vi "Rule Base Chart and Fault Probabilites Ver001.vi"(6 "s - value":dbl=1.0, 8 "Feature Thresholds":dbl[](array[numeric])=[0.583, 0.9072, 1.361, 0.43, 0.743, 0.346, 0.493], 9 "Rule Array":dbl[][](array[numeric])=[[1.0, 0.0, 1.0, -1.0, -1.0, -1.0, -1.0], [1.0, 0.0, 1.0, 1.0, -1.0, 0.0, -1.0], [-1.0, 0.0, 0.0, -1.0, 0.0, -1.0, 1.0], [-1.0, 1.0, 1.0, -1.0, 1.0, -1.0, -1.0], [0.0, 0.0, 0.0, -1.0, -1.0, -1.0, -1.0], [0.0, 0.0, 1.0, 1.0, 1.0, 0.0, 0.0], [0.0, 0.0, 0.0, 0.0, 0.0, 0.0, 0.0]], 10 "Predicted Values":dbl[](array[numeric]), 11 "Measured Values":dbl[](array[numeric])) -> (0 "Individual Probabilities (0>1)":dbl[][](array[numeric])=[[1.0, 0.0, 1.0, -1.0, -1.0, -1.0, -1.0], [1.0, 0.0, 1.0, 1.0, -1.0, 0.0, -1.0], [-1.0, 0.0, 0.0, -1.0, 0.0, -1.0, 1.0], [-1.0, 1.0, 1.0, -1.0, 1.0, -1.0, -1.0], [0.0, 0.0, 0.0, -1.0, -1.0, -1.0, -1.0], [0.0, 0.0, 1.0, 1.0, 1.0, 0.0, 0.0], [0.0, 0.0, 0.0, 0.0, 0.0, 0.0, 0.0]] format="%.2f", 1 "Fault Probability":dbl[](array[numeric]) format="%.4e", 2 "Neutral, Negative, Positive":dbl[][](array[numeric]) format="%.3e", 3 "Residuals":dbl[](array[numeric]), 4 "Individual Probabilities (%)":dbl[][](array[numeric])=[[1.0, 0.0, 1.0, -1.0, -1.0, -1.0, -1.0], [1.0, 0.0, 1.0, 1.0, -1.0, 0.0, -1.0], [-1.0, 0.0, 0.0, -1.0, 0.0, -1.0, 1.0], [-1.0, 1.0, 1.0, -1.0, 1.0, -1.0, -1.0], [0.0, 0.0, 0.0, -1.0, -1.0, -1.0, -1.0], [0.0, 0.0, 1.0, 1.0, 1.0, 0.0, 0.0], [0.0, 0.0, 0.0, 0.0, 0.0, 0.0, 0.0]] format="%.2f")   [LabVIEW 2017]
panel:
  in  "Tab Control":T1(tab)
  out "Sum of Probs":dbl[](array[numeric]) format="%_2f"
  # "Rule Based Chart"
  # "Te"
  # "Tsh"
  # "TD"
  # "Order\nfrom top\nto bottom\nas seen in\nTable 5.2 \n(Left to right)"
  # "TC"
  # "Tsc"
  # "dTCA"
  # "dTEA"
  # "Te"
  # "Tsh"
  # "TD"
  # "TC"
  # "Tsc"
  # "dTCA"
  # "dTEA"
  # "Tsh"
  # "TD"
  # "TC"
  # "Tsc"
  # "dTCA"
  # "Te"
  # "dTEA"
  # "CMF = Comp Valve Leakage"
  # "ODFoul = OD Coil Fouling"
  # "IDFoul = ID Coil Fouling"
  # "LL = Liq. Line Restriction"
  # "UC = Undercharge (- %)"
  # "OC = Overcharge (+ %)"
  # "NF = No Fault"
  # "Te"
  # "Tsh"
  # "TD"
  # "TC"
  # "Tsc"
  # "dTCA"
  # "dTEA"
  # "0"
  # "-1"
  # "1"
  # "CMF = Comp Valve Leakage"
  # "ODFoul = OD Coil Fouling"
  # "IDFoul = ID Coil Fouling"
  # "LL = Liq. Line Restriction"
  # "UC = Undercharge (- %)"
  # "OC = Overcharge (+ %)"
  # "NF = No Fault"
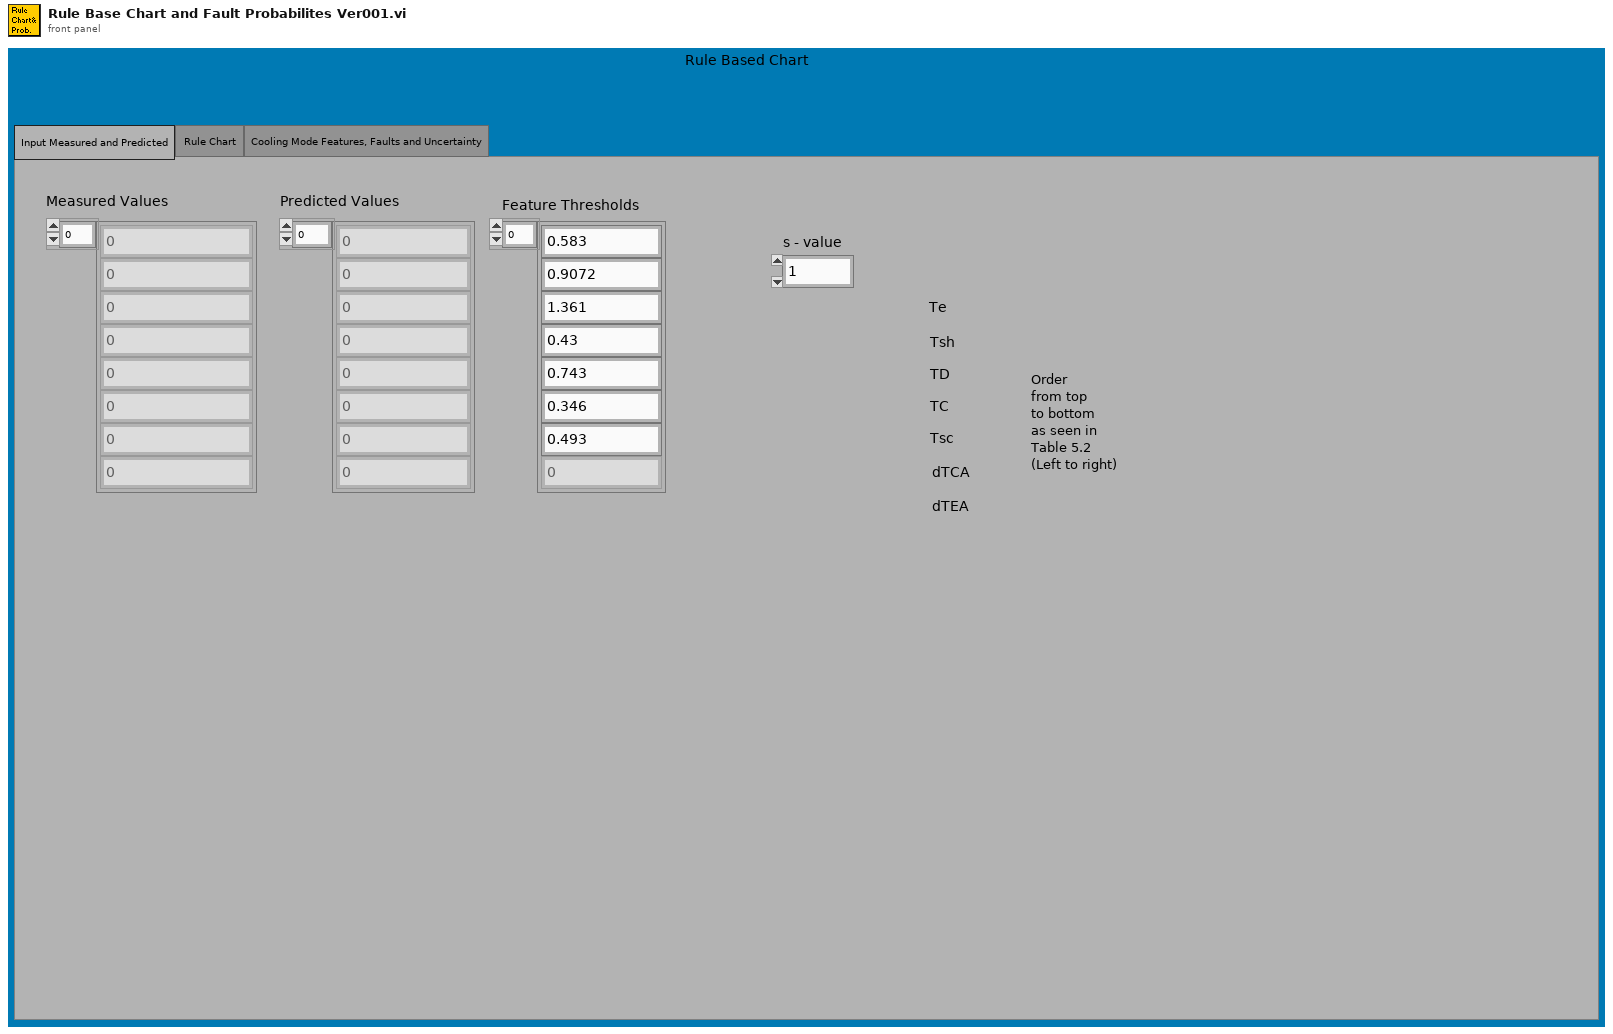
[diagram p1: front panel]
types:
  T1 = enum32{"Input Measured and Predicted", "Rule Chart ", "Cooling Mode Features, Faults and Uncertainty"}
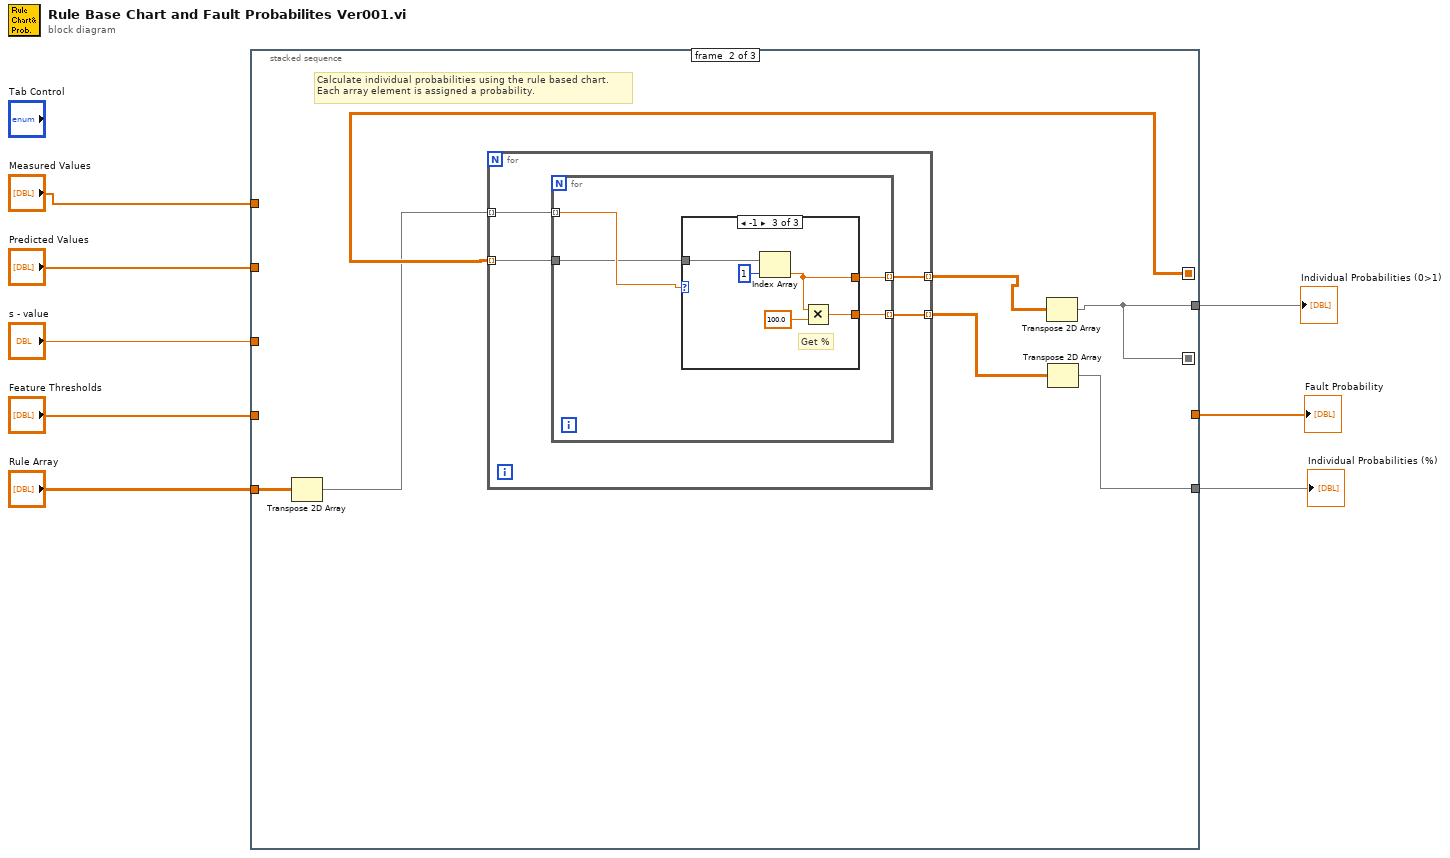
[diagram p0: block diagram]
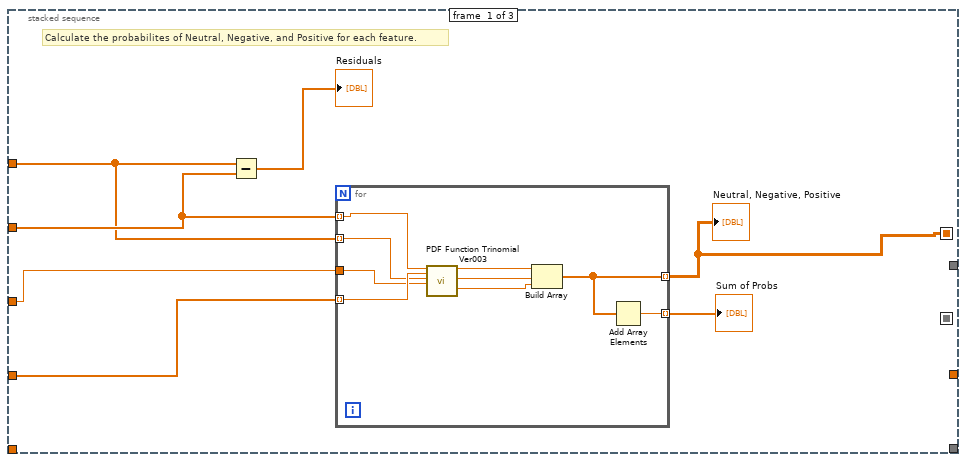
[diagram p2: hidden frame]
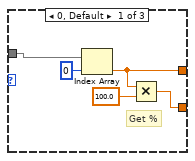
[diagram p3: hidden frame]
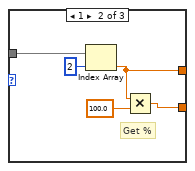
[diagram p4: hidden frame]
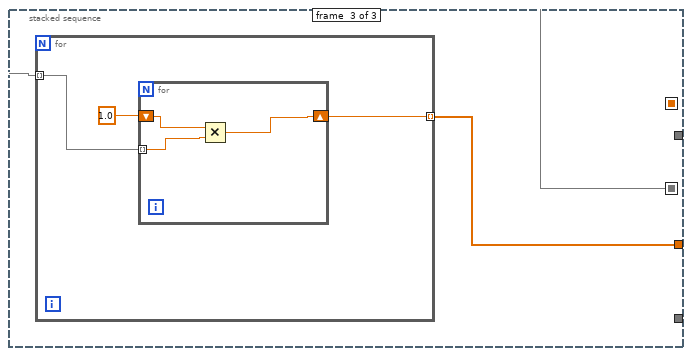
[diagram p5: hidden frame]
diagram:
  n1 = stacked-sequence {
    seq-local: [w9 _ _] -> [_ w31 _]
    seq-local: [_ w27 _] -> [_ _ w56]
    tunnel: "Measured Values" -> [w13 _ _]
    tunnel: "Predicted Values" -> [w14 _ _]
    tunnel: "s - value" -> [w12 _ _]
    tunnel: "Feature Thresholds" -> [w11 _ _]
    tunnel: "Rule Array" -> [_ w30 _]
    tunnel: [_ w27 _] -> w3
    tunnel: [_ _ w55] -> w2
    tunnel: [_ w25 _] -> w1
    frame #0 {
      # "Calculate the probabilites of Neutral, Negative, and Positive for each feature."
      n2 = Subtract(x=w13, y=w14) -> (x-y=→"Residuals":dbl[])
      n3 = for {
        tunnel: w14 -> [w24] mode=indexing
        tunnel: w13 -> [w22] mode=indexing
        tunnel: w12 -> [w21]
        tunnel: w11 -> [w23] mode=indexing
        tunnel: [w17] -> w9 mode=indexing
        tunnel: [w16] -> w10 mode=indexing
        n4 = call "PDF Function Trinomial Ver003.vi"("NFSS Ref \nModel Value"=w24, "NFSS Ref Std Dev"=w23, "Current Measured Value\nor Moving Window Mean"=w22, "s - value"=w21) -> ("Probability of NEUTRAL"=w20:dbl, "Prob NEGATIVE\nor DECREASING"=w19:dbl, "Prob POSITIVE\nor INCREASING"=w18:dbl)  [unwired: 13 out]
        n5 = Build Array(w20, w19, w18) -> (w17:dbl[])
        n6 = Add Array Elements(numeric array=w17) -> (sum=w16:dbl)
      }
      "Neutral, Negative, Positive" <- w9
      "Sum of Probs" <- w10
    }
    frame #1 {
      # "Calculate individual probabilities using the rule based chart.\nEach array element is assigned a probability."
      n7 = Transpose 2D Array(2D array=w30) -> (transposed array=w29:dbl[][])
      n8 = for {
        tunnel: w29 -> [w35] mode=indexing
        tunnel: w31 -> [w34] mode=indexing
        tunnel: [w33] -> w28 mode=indexing
        tunnel: [w32] -> w26 mode=indexing
        n9 = for {
          tunnel: w35 -> [w39] mode=indexing
          tunnel: w34 -> [w38]
          tunnel: [w37] -> w33 mode=indexing
          tunnel: [w36] -> w32 mode=indexing
          n10 = case shown="-1" w39 {
            tunnel: w38 -> [w44 w48 w53]
            tunnel: [w41 w46 w51] -> w37
            tunnel: [w40 w45 w50] -> w36
            frame 0, Default {
              # "Get %"
              n11 = Index Array(array=w44, index=0) -> (element=w41:dbl)
              n12 = Multiply(x=w41, y=100.0) -> (x*y=w40:dbl)
            }
            frame 1 {
              # "Get %"
              n13 = Index Array(array=w48, index=2) -> (element=w46:dbl)
              n14 = Multiply(x=w46, y=100.0) -> (x*y=w45:dbl)
            }
            frame -1 {
              # "Get %"
              n15 = Index Array(array=w53, index=1) -> (element=w51:dbl)
              n16 = Multiply(x=w51, y=100.0) -> (x*y=w50:dbl)
            }
          }
        }
      }
      n17 = Transpose 2D Array(2D array=w28) -> (transposed array=w27:dbl[][])
      n18 = Transpose 2D Array(2D array=w26) -> (transposed array=w25:dbl[][])
    }
    frame #2 {
      n19 = for {
        tunnel: w56 -> [w58] mode=indexing
        tunnel: [w57] -> w55 mode=indexing
        n20 = for {
          shift-right: [w60] -> w57
          shift-left: 1.0 -> [w62]
          tunnel: w58 -> [w61] mode=indexing
          n21 = Multiply(x=w62, y=w61) -> (x*y=w60:dbl)
        }
      }
    }
  }
  "Individual Probabilities (0>1)" <- w3
  "Fault Probability" <- w2
  "Individual Probabilities (%)" <- w1
